vi "Launch HW Info.vi"(8 "error in (no error)":errorcluster, 11 "Volatus Core in":refnum<class "Volatus Core.lvclass">) -> (0 "error out":errorcluster, 3 "Volatus Core out":refnum<class "Volatus Core.lvclass">)   [LabVIEW 2020, in "Volatus.lvlib" / "Volatus Core.lvclass"]
uses:
  Volatus Core.lvclass
  C:/dev/lv20CE/relink/lv-volatus/Volatus/Module/Module.lvclass
  Hardware Info Module/Hardware Info Module.lvclass
  VolatusConfig/VolatusConfigElement/VolatusConfigElement.lvclass
  Volatus Core.lvclass/Volatus Core.ctl
  Module/Module.lvclass
  C:/dev/lv20CE/relink/lv-volatus/Volatus/Hardware Info Module/Hardware Info Module.lvclass
  C:/dev/lv20CE/relink/lv-volatus/Volatus/Volatus Core/Volatus Core.lvclass
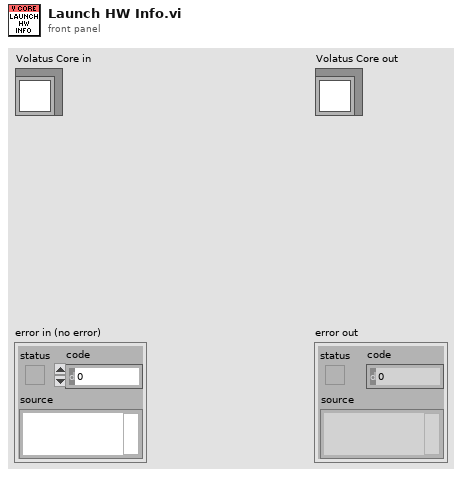
[diagram p1: front panel]
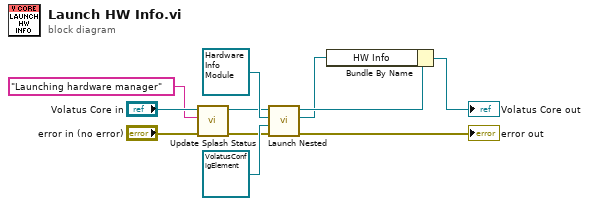
[diagram p0: block diagram]
diagram:
  n1 = call "Update Splash Status.vi"("error in (no error)"="error in (no error)", "Status"="Launching hardware manager", "Volatus Core in"="Volatus Core in") -> ("error out"=w4:errorcluster, "Volatus Core out"=w2:refnum<class "Volatus Core.lvclass">)  [unwired: 7 in]
  n2 = call "Launch Nested.vi"("error in (no error)"=w4, "Config Element"=refnum<class "VolatusConfigElement.lvclass"> refnum, "Nested Module"=refnum<class "Hardware Info Module.lvclass"> refnum ("Volatus:Hardware Info Module.lvclass"), "Parent in"=w2) -> ("error out"=→"error out":errorcluster, "MessageQ"=w5:refnum<class "MessageQ.lvclass">, "Parent out"=w9:refnum<class "Volatus Core.lvclass">)  [unwired: 5 in]
  n3 = Bundle By Name(cluster=w9, "HW Info"=w5) -> (→"Volatus Core out":refnum<class "Volatus Core.lvclass">)
